vi "LoadAllControls.vi"(8 "error in (no error)":errorcluster, 10 "menu reference":refnum<k9>, 11 "This VI":refnum<vi>) -> (0 "error out":errorcluster, 3 "FP Controls out":refnum<class "FP Controls.lvclass">)   [LabVIEW 2012, in "Configuration Grandmaster.lvlib" / "FP Controls.lvclass"]
uses:
  FP Controls.lvclass
  Common/Controls/Group Timing Info.ctl
  Common/Controls/LS Lock Sizes.ctl
  FP Controls.lvclass/FP Controls.ctl
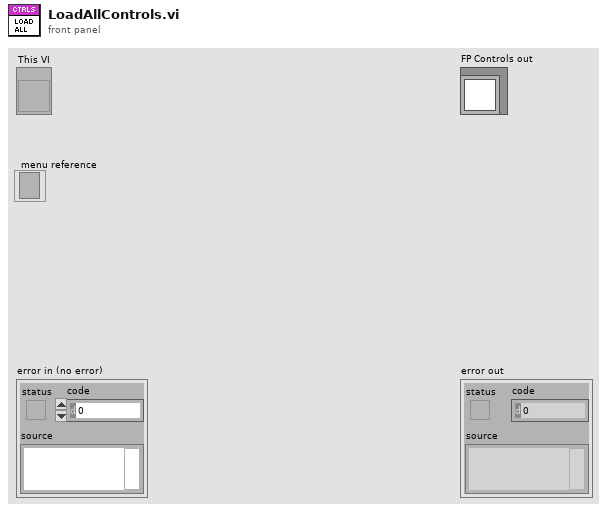
[diagram p1: front panel]
types:
  T1 = typedef "LS Lock Sizes.ctl" = enum16{"No", "250ms", "500ms", "1s"}
  T2 = typedef "Group Timing Info.ctl" = cluster{"Rate":dbl, "ReadBlk":i32}
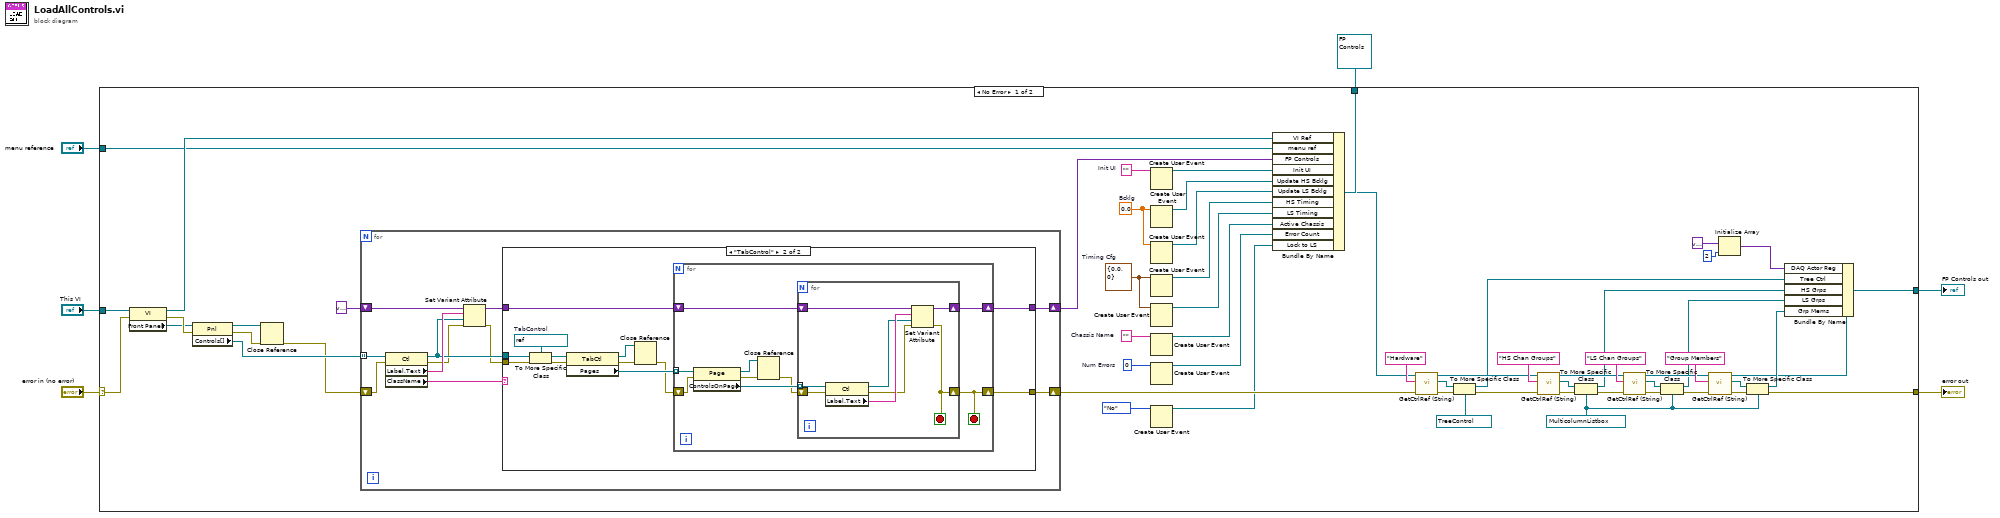
[diagram p0: block diagram]
diagram:
  n1 = case shown="No Error" "error in (no error)" {
    selector: "error in (no error)" -> [w60 w109]
    tunnel: [w34 w109] -> w5
    tunnel: "This VI" -> [w61 _]
    tunnel: refnum<class "FP Controls.lvclass"> refnum ("FP Controls out") -> [w56 w108]
    tunnel: [w25 w108] -> w2
    tunnel: "menu reference" -> [w53 _]
    frame No Error {
      w15 = 0.0  # Bcklg
      w18 = u32 0  # Num Errors
      w20 = ""  # Chassis Name
      w27 = refnum<vi> refnum ("HS Chan Groups")
      w50 = T2 {"Rate"=0.0, "ReadBlk"=0}  # Timing Cfg
      w52 = ""  # Init UI
      n2 = property class="VI"(reference=w61, error in=w60) -> (reference out=w55:refnum<vi>, error out=w65:errorcluster, "Front Panel"=w64:refnum<vi>)
      n3 = property class="Pnl"(reference=w64, error in=w65) -> (reference out=w62:refnum<vi>, error out=w63:errorcluster, "Controls[]"=w59:refnum<vi>[])
      n4 = Close Reference(reference=w62, error in (no error)=w63) -> (error out=w54:errorcluster)
      n5 = for {
        tunnel: w59 -> [w76] mode=indexing
        shift-right: [w68] -> w57
        shift-left: variant ("FP Controls") -> [w74]
        shift-right: [w67] -> w48
        shift-left: w54 -> [w75]
        n6 = property class="Ctl"(reference=w76, error in=w75) -> (reference out=w72:refnum<vi>, error out=w71:errorcluster, "Label.Text"=w73:string, "ClassName"=w66:string)
        n7 = Set Variant Attribute(Variant=w74, name=w73, value=w72, error in=w71) -> (Variant out=w69:variant, error out=w70:errorcluster)  [unwired: 1 out]
        n8 = case shown="\"TabControl\"" w66 {
          tunnel: w72 -> [_ w82]
          tunnel: w70 -> [w77 w83]
          tunnel: w69 -> [w78 w81]
          tunnel: [w78 w80] -> w68
          tunnel: [w77 w79] -> w67
          frame Default {
          }
          frame "TabControl" {
            w88 = refnum<vi> refnum  # TabControl
            n9 = To More Specific Class(target class=w88, reference=w82, error in=w83) -> (specific class reference=w89:refnum<vi>, error out=w90:errorcluster)
            n10 = property class="TabCtl"(reference=w89, error in=w90) -> (reference out=w86:refnum<vi>, error out=w87:errorcluster, "Pages"=w85:refnum<vi>[])
            n11 = Close Reference(reference=w86, error in (no error)=w87) -> (error out=w84:errorcluster)
            n12 = for {
              tunnel: w85 -> [w97] mode=indexing
              shift-right: [w91] -> w79
              shift-left: w84 -> [w96]
              shift-right: [w92] -> w80
              shift-left: w81 -> [w93]
              stop <- w91 stop-if-true
              n13 = property class="Page"(reference=w97, error in=w96) -> (reference out=w99:refnum<vi>, error out=w98:errorcluster, "ControlsOnPage"=w95:refnum<vi>[])
              n14 = Close Reference(reference=w99, error in (no error)=w98) -> (error out=w94:errorcluster)
              n15 = for {
                tunnel: w95 -> [w107] mode=indexing
                shift-right: [w100] -> w91
                shift-left: w94 -> [w106]
                shift-right: [w105] -> w92
                shift-left: w93 -> [w104]
                stop <- w100 stop-if-true
                n16 = property class="Ctl"(reference=w107, error in=w106) -> (reference out=w102:refnum<vi>, error out=w101:errorcluster, "Label.Text"=w103:string)
                n17 = Set Variant Attribute(Variant=w104, name=w103, value=w102, error in=w101) -> (Variant out=w105:variant, error out=w100:errorcluster)  [unwired: 1 out]
              }
            }
          }
        }
      }
      n18 = Create User Event(user event datatype=w52) -> (user event=w51:refnum<user-event>)  [unwired: 1 in, 1 out]
      n19 = Create User Event(user event datatype=w15) -> (user event=w14:refnum<user-event>)  [unwired: 1 in, 1 out]
      n20 = Create User Event(user event datatype=w15) -> (user event=w13:refnum<user-event>)  [unwired: 1 in, 1 out]
      n21 = Create User Event(user event datatype=w50) -> (user event=w16:refnum<user-event>)  [unwired: 1 in, 1 out]
      n22 = Create User Event(user event datatype=w50) -> (user event=w49:refnum<user-event>)  [unwired: 1 in, 1 out]
      n23 = Create User Event(user event datatype=w20) -> (user event=w19:refnum<user-event>)  [unwired: 1 in, 1 out]
      n24 = Create User Event(user event datatype=w18) -> (user event=w17:refnum<user-event>)  [unwired: 1 in, 1 out]
      n25 = Create User Event(user event datatype=LS_Lock_Sizes."No" ("GlobalBlockSize")) -> (user event=w7:refnum<user-event>)  [unwired: 1 in, 1 out]
      n26 = Bundle By Name(cluster=w56, "VI Ref"=w55, "menu ref"=w53, "FP Controls"=w57, "Init UI"=w51, "Update HS Bcklg"=w14, "Update LS Bcklg"=w13, "HS Timing"=w16, "LS Timing"=w49, "Active Chassis"=w19, "Error Count"=w17, "Lock to LS"=w7) -> (w26:refnum<class "FP Controls.lvclass">)
      n27 = call "GetCtrlRef (String).vi"("error in (no error)"=w48, "FP Control"="Hardware", "FP Controls in"=w26) -> ("error out"=w46:errorcluster, "Ctrl Ref"=w47:refnum<vi>, "FP Controls out"=w30:refnum<class "FP Controls.lvclass">)  [unwired: 6 in]
      n28 = To More Specific Class(target class=refnum<vi> refnum ("Hardware"), reference=w47, error in=w46) -> (specific class reference=w24:refnum<vi>, error out=w45:errorcluster)
      n29 = call "GetCtrlRef (String).vi"("error in (no error)"=w45, "FP Control"="HS Chan Groups", "FP Controls in"=w30) -> ("error out"=w35:errorcluster, "Ctrl Ref"=w33:refnum<vi>, "FP Controls out"=w29:refnum<class "FP Controls.lvclass">)  [unwired: 6 in]
      n30 = To More Specific Class(target class=w27, reference=w33, error in=w35) -> (specific class reference=w23:refnum<vi>, error out=w36:errorcluster)
      n31 = call "GetCtrlRef (String).vi"("error in (no error)"=w36, "FP Control"="LS Chan Groups", "FP Controls in"=w29) -> ("error out"=w43:errorcluster, "Ctrl Ref"=w32:refnum<vi>, "FP Controls out"=w28:refnum<class "FP Controls.lvclass">)  [unwired: 6 in]
      n32 = To More Specific Class(target class=w27, reference=w32, error in=w43) -> (specific class reference=w22:refnum<vi>, error out=w37:errorcluster)
      n33 = call "GetCtrlRef (String).vi"("error in (no error)"=w37, "FP Control"="Group Members", "FP Controls in"=w28) -> ("error out"=w42:errorcluster, "Ctrl Ref"=w31:refnum<vi>, "FP Controls out"=w12:refnum<class "FP Controls.lvclass">)  [unwired: 6 in]
      n34 = Initialize Array(variant ("FP Controls"), 2 ("dimension size")) -> (w11:variant[])
      n35 = To More Specific Class(target class=w27, reference=w31, error in=w42) -> (specific class reference=w21:refnum<vi>, error out=w34:errorcluster)
      n36 = Bundle By Name(cluster=w12, "DAQ Actor Reg"=w11, "Tree Ctrl"=w24, "HS Grps"=w23, "LS Grps"=w22, "Grp Mems"=w21) -> (w25:refnum<class "FP Controls.lvclass">)
    }
    frame Error {
    }
  }
  "error out" <- w5
  "FP Controls out" <- w2
